vi "Test Real-Time Camera.vi"() -> ()   [LabVIEW 2014]
uses:
  vi.lib/Q-WaveSystems/QwaveSys Raspberry Pi for LabVIEW Home-Education/QwaveSys Raspberry Pi Library.lvlib
panel:
  in  "camnum":i32
  out "h":i32
  out "w":i32
  in  "stop":bool
  out "return type 2":i32
  out "return type":i32
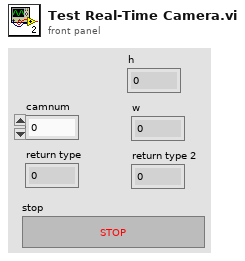
[diagram p1: front panel]
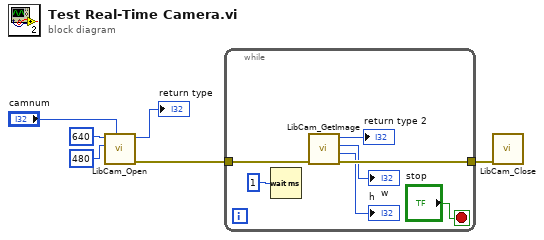
[diagram p0: block diagram]
diagram:
  n1 = call "LibCam_Open.vi"("webcamnum"="camnum", "height"=480 ("h"), "width"=640 ("w")) -> ("error out"=w2:errorcluster, "return type"=→"return type":i32)  [unwired: 7 in]
  n2 = while {
    tunnel: [w11] -> w1
    tunnel: w2 -> [w9]
    stop <- "stop" stop-if-true
    n3 = Wait (ms)(milliseconds to wait=u32 1) -> ()  [unwired: 1 out]
    n4 = call "LibCam_GetImage.vi"("error in (no error)"=w9) -> ("error out"=w11:errorcluster, "height"=→"h":i32, "width"=→"w":i32, "return type"=→"return type 2":i32)  [unwired: 7 in]
  }
  n5 = call "LibCam_Close.vi"("error in (no error)"=w1) -> ()  [unwired: 10 in, 1 out]
